vi "CCC Example - Server.vi"() -> ()   [LabVIEW 2010]
doc: "This VI shows an example of how to use the CVT Client Communication API. This VI is meant to be used in conjunction with \"CCC Client Example.vi\"."
uses:
  <vilib>/NI/Current Value Table/Type Defs/Single Tag.ctl
  <vilib>/NI/Current Value Table/Type Defs/Data Types.ctl
  <vilib>/NI/Current Value Table/Type Defs/File Format.ctl
  <vilib>/NI/Current Value Table/Type Defs/Tag Grouping set.ctl
  <vilib>/NI/Current Value Table/DataTypes/Double_Read.vi
  <vilib>/NI/Current Value Table/DataTypes/String_Read.vi
  <vilib>/NI/Current Value Table/DataTypes/Double_Write.vi
  <vilib>/NI/Current Value Table/DataTypes/Boolean_Write.vi
  <vilib>/NI/Current Value Table/Type to Enum.vi
  <vilib>/NI/Current Value Table/DataTypes/Double_Type To Enum.vi
  <vilib>/NI/Current Value Table/DataTypes/String_Type To Enum.vi
  <vilib>/NI/Current Value Table/DataTypes/Boolean_Type To Enum.vi
  <vilib>/NI/Current Value Table/FGVs/CVT Globals.vi
  <vilib>/NI/Current Value Table/FGVs/Tag Memory.vi
  <vilib>/NI/Current Value Table/Memory Block.vi
  <vilib>/NI/Current Value Table/DataTypes/Double_Memory Block.vi
  <vilib>/NI/Current Value Table/DataTypes/String_Memory Block.vi
  <vilib>/NI/Current Value Table/DataTypes/Boolean_Memory Block.vi
  vi.lib/NI/CCC/NI_CCC.lvlib
  <vilib>/NI/Current Value Table/Current Value Table.lvlib
panel:
  in  "CVT Tags":T1[](array[typedef])=[{"Data Type"=enum."Double", "Name"="Float1", "Value"="", "Description"=""}, {"Data Type"=enum."Double", "Name"="Float2", "Value"="", "Description"=""}, {"Data Type"=enum."Double", "Name"="Float3", "Value"="", "Description"=""}, {"Data Type"=enum."String", "Name"="Operand", "Value"="", "Description"=""}, {"Data Type"=enum."Boolean", "Name"="Error", "Value"="", "Description"=""}]
  out "error out":errorcluster
  in  "stop":bool
  # "Directions:\nRun this VI first, followed by \"CCC Example - Client.vi\""
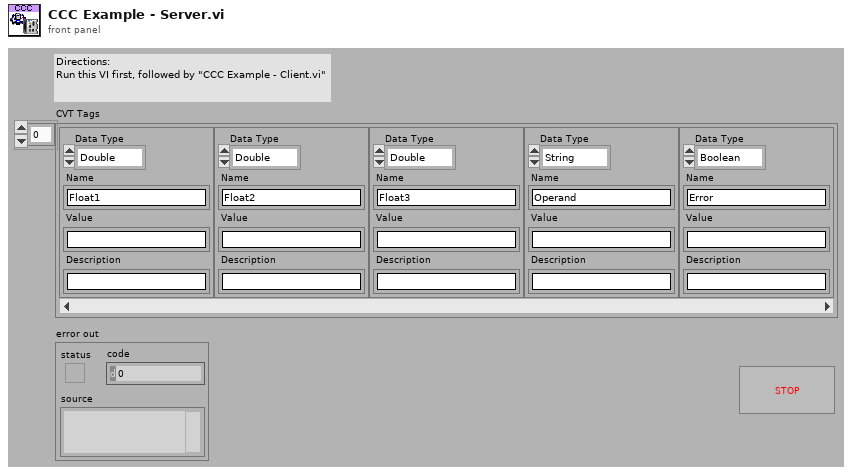
[diagram p1: front panel]
types:
  T1 = typedef "Current Value Table.lvlib/Single Tag.ctl" = cluster{"Data Type":T2, "Name":string, "Value":string, "Description":string}
  T2 = typedef "Current Value Table.lvlib/Data Types.ctl" = enum16{"Double", "Single", "I64", "I32", "I16", "I8", "U64", "U32", "U16", "U8", "String", "Boolean", "Array of U8", "Array of U16", "Array of U32", "Array of U64", "Array of I64", "Array of I32", "Array of I16", "Array of I8", "Array of Double", "Array of Single", "Array of Boolean", "Array of String"}
  T3 = typedef "Current Value Table.lvlib/File Format.ctl" = cluster{"Tags":T1[], "Group Listings":T4[]}
  T4 = typedef "Current Value Table.lvlib/Tag Grouping set.ctl" = cluster{"Group":string, "Tag Names":string[]}
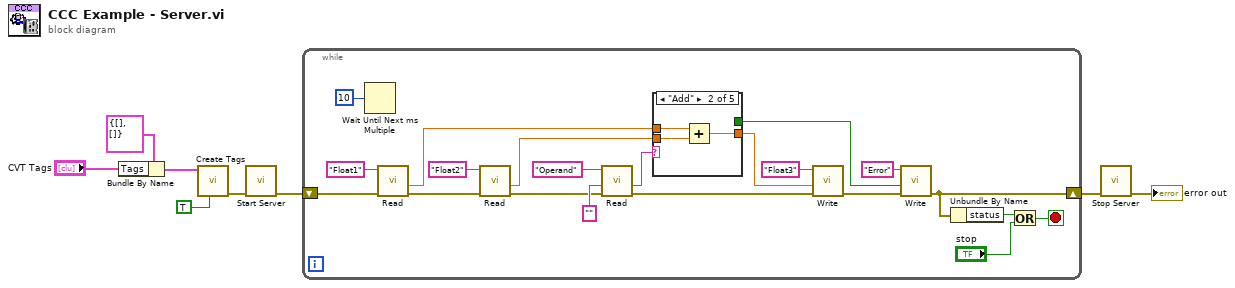
[diagram p0: block diagram]
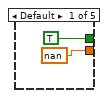
[diagram p2: hidden frame]
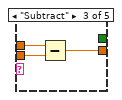
[diagram p3: hidden frame]
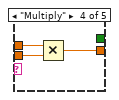
[diagram p4: hidden frame]
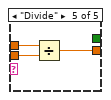
[diagram p5: hidden frame]
diagram:
  n1 = Bundle By Name(cluster=T3 {"Tags"=[], "Group Listings"=[]} ("CVT Tags to Create"), "Tags"="CVT Tags") -> (w2:T3)
  n2 = call <vilib>:"Create Tags.vi"("Overwrite Duplicates? (F)"=TRUE ("Clear Table? (F)"), "CVT Tags to Create"=w2) -> ("error out"=w8:errorcluster)  [unwired: 9 in]
  n3 = call "Start Server.vi"("error in"=w8) -> ("error out"=w7:errorcluster)  [unwired: 10 in]
  n4 = while {
    shift-right: [w12] -> w6
    shift-left: w7 -> [w13]
    stop <- w10 stop-if-true
    n5 = Wait Until Next ms Multiple(millisecond multiple=u32 10) -> ()  [unwired: 1 out]
    n6 = call-poly <vilib>:"Read.vi"("error in (no error)"=w13, "Tag Name"="Float1") -> ("error out"=w17:errorcluster, "Value"=w28:dbl)  [unwired: 8 in]
    n7 = call-poly <vilib>:"Read.vi"("error in (no error)"=w17, "Tag Name"="Float2") -> ("error out"=w16:errorcluster, "Value"=w25:dbl)  [unwired: 8 in]
    n8 = call-poly <vilib>:"Read.vi"("error in (no error)"=w16, "Default"="", "Tag Name"="Operand") -> ("error out"=w15:errorcluster, "Value"=w23:string)  [unwired: 7 in]
    n9 = case shown="\"Add\"" w23 {
      tunnel: w28 -> [_ w34 w37 w40 w43]
      tunnel: w25 -> [_ w33 w36 w39 w42]
      tunnel: [nan w32 w35 w38 w41] -> w20
      tunnel: [TRUE ("stop") _ _ _ _] -> w18
      frame Default {
      }
      frame "Add" {
        n10 = Add(x=w34, y=w33) -> (x+y=w32:dbl)
      }
      frame "Subtract" {
        n11 = Subtract(x=w37, y=w36) -> (x-y=w35:dbl)
      }
      frame "Multiply" {
        n12 = Multiply(x=w40, y=w39) -> (x*y=w38:dbl)
      }
      frame "Divide" {
        n13 = Divide(x=w43, y=w42) -> (x/y=w41:dbl)
      }
    }
    n14 = call-poly <vilib>:"Write.vi"("error in (no error)"=w15, "Value"=w20, "Tag Name"="Float3") -> ("error out"=w14:errorcluster)  [unwired: 8 in]
    n15 = call-poly <vilib>:"Write.vi"("error in (no error)"=w14, "Value"=w18, "Tag Name"="Error") -> ("error out"=w12:errorcluster)  [unwired: 8 in]
    n16 = Unbundle By Name(w12) -> ("status"=w11:bool)
    n17 = Or(x=w11, y="stop") -> (x .or. y?=w10:bool)
  }
  n18 = call "Stop Server.vi"("error in"=w6) -> ("error out"=→"error out":errorcluster)  [unwired: 10 in]
